vi "Player Info.vi"(8 "Victory Speech":string="Victory is mine!!!", 9 "Name":string="Wanderer", 11 "Wanderer in":refnum<class "Wanderer.lvclass">) -> (3 "Wanderer out":refnum<class "Wanderer.lvclass">)   [LabVIEW 2015, in "Wanderer.lvclass"]
uses:
  Wanderer.lvclass
  Square/Square.lvclass
panel:
  # "Set default values for these two string controls"
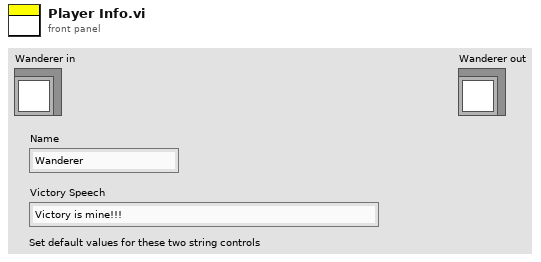
[diagram p1: front panel]
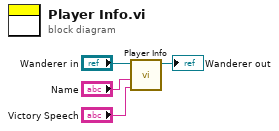
[diagram p0: block diagram]
diagram:
  n1 = call-parent "Player Info.vi"("Victory Speech"="Victory Speech", "Name"="Name", "Square in"="Wanderer in") -> ("Square out"=→"Wanderer out":refnum<class "Wanderer.lvclass">)  [unwired: 8 in]
